vi "Change IP test.vi"() -> ()   [LabVIEW 2021]
uses:
  Ethernet/Ethernet.lvclass
panel:
  in  "UDP port":u16=54321
  in  "TCP port":u16=12345
  in  "Box IP address":string="192.168.1.100"
  in  "new IP Address":string
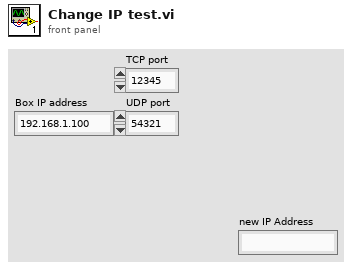
[diagram p1: front panel]
types:
  T1 = typedef "Battery Simulator 1200 LabVIEW Driver.lvlib/Ethernet.lvclass/Ethernet Settings.ctl" = cluster{"IP Address":string, "TCP (Command) Port":u16, "TCP (Command) Read Interval (ms)":u32, "UDP (Reporting) Port":u16, "UDP (Reporting) Write Interval (ms)":u32}
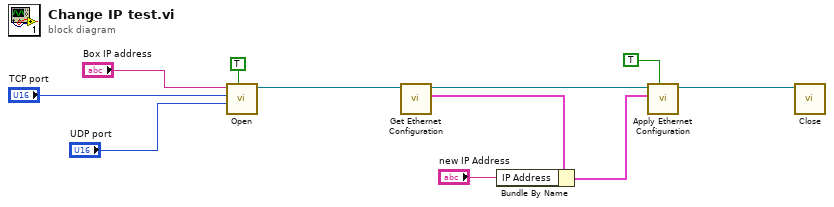
[diagram p0: block diagram]
diagram:
  n1 = call "Open.vi"("Connect for Config Only? (F)"=TRUE, "UDP port"="UDP port", "TCP port"="TCP port", "Box IP address"="Box IP address") -> ("ENET out"=w10:refnum<class "Ethernet.lvclass">)  [unwired: 6 in, 1 out]
  n2 = call "Get Ethernet Configuration.vi"("Ethernet in"=w10) -> ("Ethernet Settings"=w8:T1, "Ethernet out"=w9:refnum<class "Ethernet.lvclass">)  [unwired: 7 in, 2 out]
  n3 = Bundle By Name(cluster=w8, "IP Address"="new IP Address") -> (w7:T1)
  n4 = call "Apply Ethernet Configuration.vi"("Restart (T)"=TRUE, "Ethernet Settings"=w7, "Ethernet in"=w9) -> ("Ethernet out"=w5:refnum<class "Ethernet.lvclass">)  [unwired: 7 in, 1 out]
  n5 = call-dynamic "Close.vi"("ENET in"=w5) -> ()  [unwired: 10 in, 1 out]
